vi "calculator.vi"() -> ()   [LabVIEW 2014]
panel:
  in  "stop":bool
  out "String":string
  in  "Cluster":T1
  # "physical keyborad位置設計的有些複雜\n\nF1對應數字鍵1\nF2對應數字鍵2\nF3對應數字鍵3\nF4對應數字鍵4\nF5對應數字鍵5\nF6對應數字鍵6\nF7對應數字鍵7\nF8對應數字鍵8\nF9對應數字鍵9\nF10對應數字鍵0\nF11對符號 . \nPGUP對應加號\nPGON對應減號\nHOME對應乘號\nEND對應除號\nDELETE對應Clear\nENTER對應等號\n\n備註:我使用MSI筆電，按加減乘除時，需搭配shift並按設定鍵兩下才有效果"
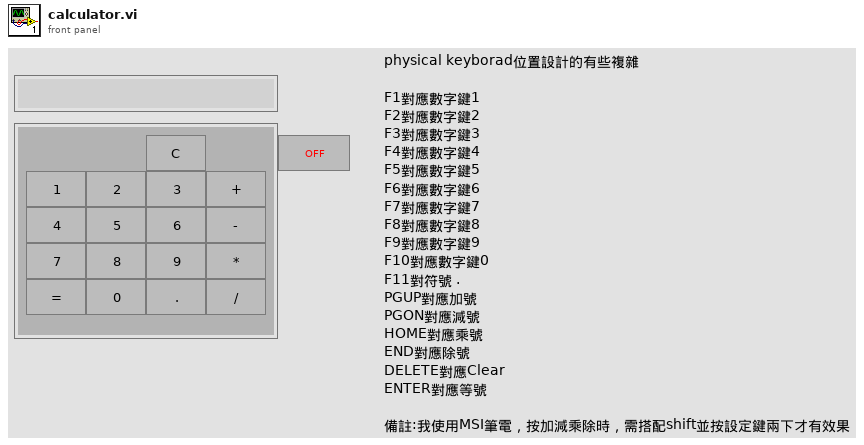
[diagram p1: front panel]
types:
  T1 = cluster{"1":bool, "2":bool, "3":bool, "4":bool, "5":bool, "6":bool, "7":bool, "8":bool, "9":bool, "0":bool, ".":bool, "add":bool, "sub":bool, "mul":bool, "div":bool, "equal":bool, "C":bool}
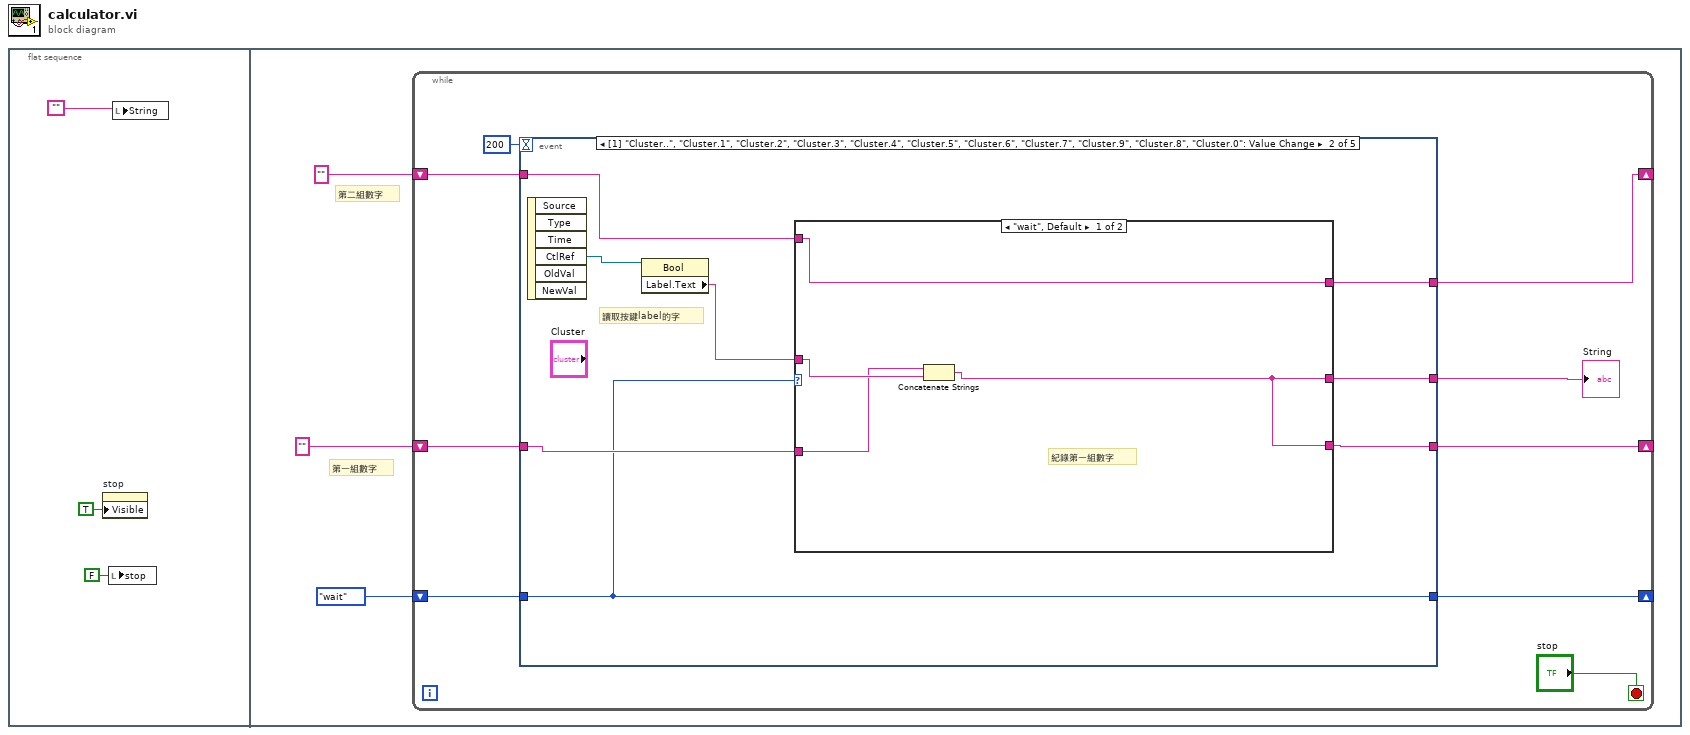
[diagram p0: block diagram]
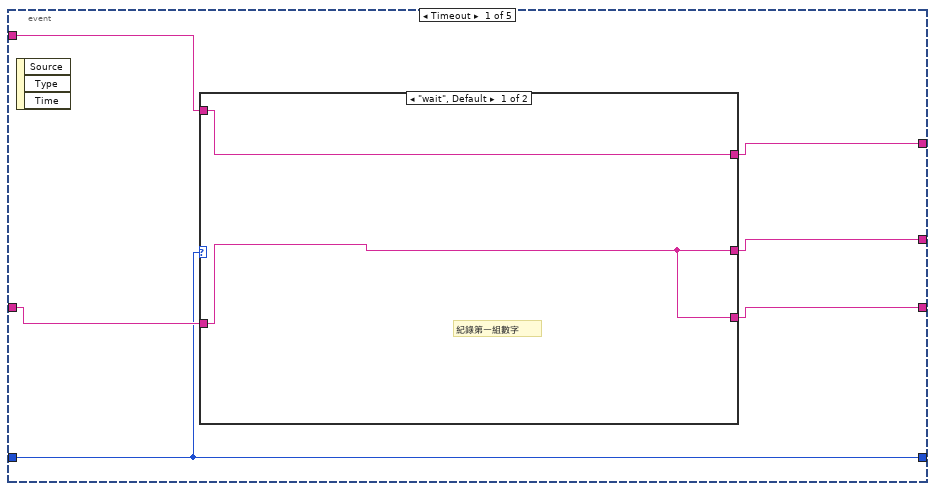
[diagram p2: hidden frame]
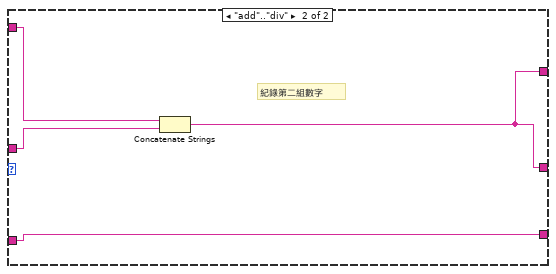
[diagram p4: hidden frame]
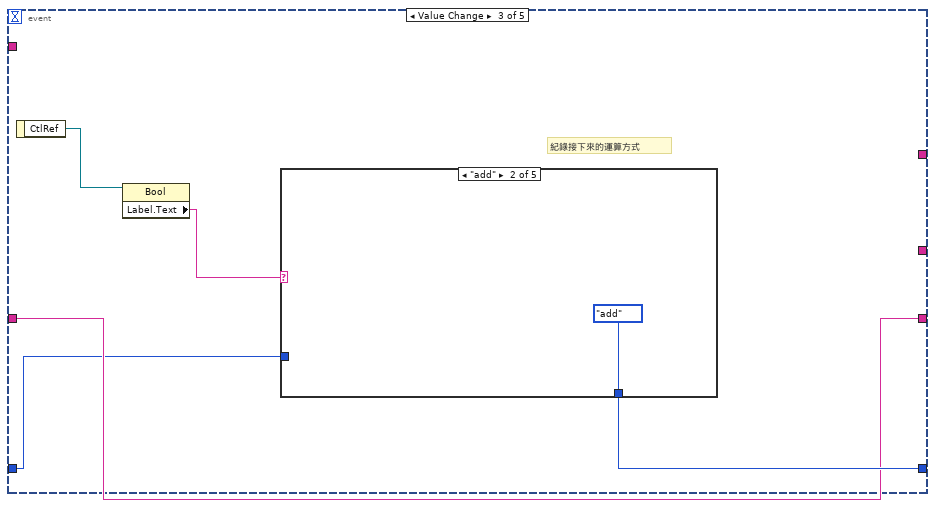
[diagram p5: hidden frame]
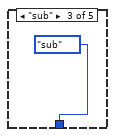
[diagram p7: hidden frame]
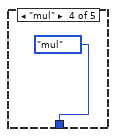
[diagram p8: hidden frame]
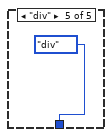
[diagram p9: hidden frame]
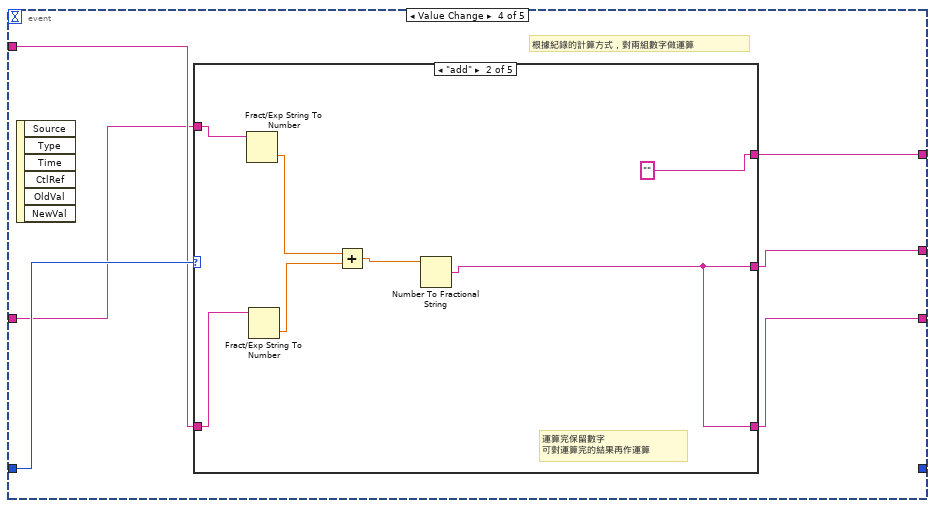
[diagram p10: hidden frame]
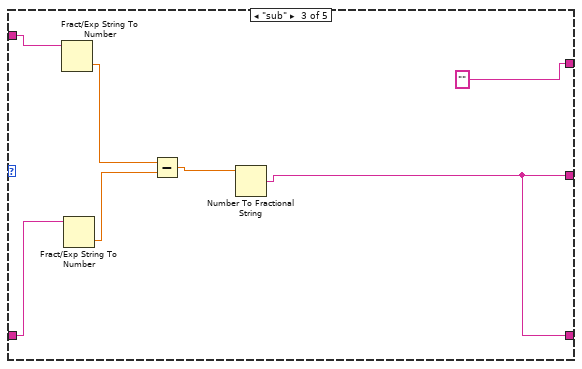
[diagram p12: hidden frame]
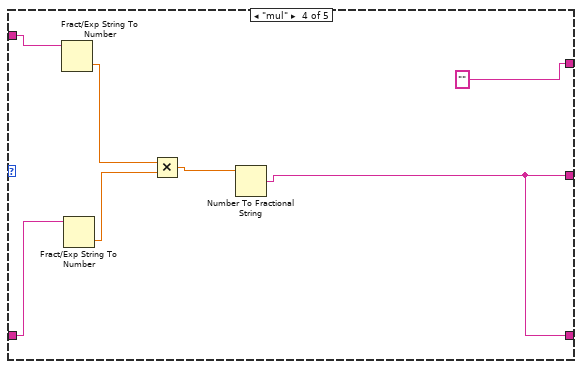
[diagram p13: hidden frame]
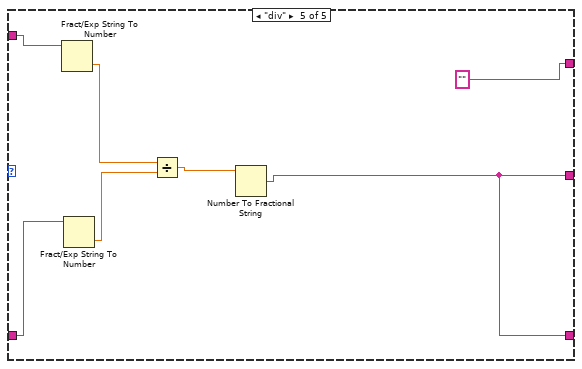
[diagram p14: hidden frame]
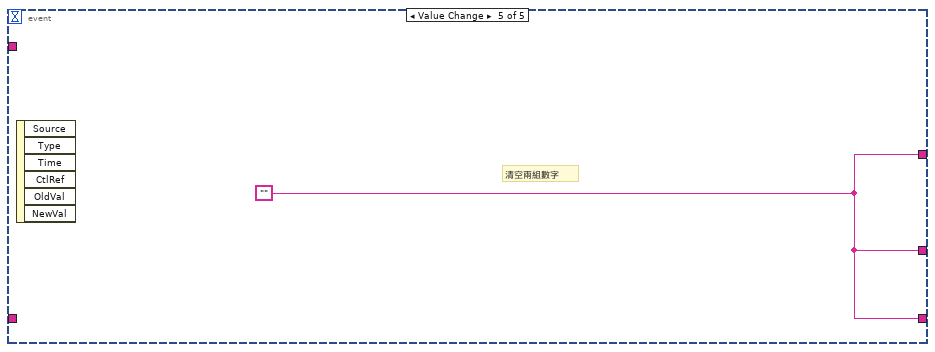
[diagram p15: hidden frame]
diagram:
  n1 = flat-sequence {
    frame #0 {
      n2 = property on="stop" class="Bool (strict)"("Visible"=TRUE) -> ()  [unwired: 2 in, 2 out]
      n3 = local write "stop"(FALSE ("stop")) -> ()
      n4 = local write "String"("") -> ()
    }
    frame #1 {
      # "第二組數字"
      # "第一組數字"
      n5 = while {
        shift-right: [w11] -> _
        shift-left: "" -> [w15]
        shift-right: [w8] -> _
        shift-left: "" -> [w14]
        shift-right: [w12] -> _
        shift-left: enum16{"wait", "add", "sub", "mul", "div"}."wait" -> [w13]
        stop <- "stop" stop-if-true
        n6 = event shown="[1] \"Cluster..\", \"Cluster.1\", \"Cluster.2\", \"Cluster.3\", \"Cluster.4\", \"Cluster.5\", \"Cluster.6\", \"Cluster.7\", \"Cluster.9\", \"Cluster.8\", \"Cluster.0\": Value Change" {
          selector: _ -> [_ _ _ _ _]
          dyn-events: _ -> [_ _ _ _ _]
          timeout: 200 -> [_ _ _ _ _]
          tunnel: w15 -> [w17 w33 _ w53 _]
          tunnel: w14 -> [w21 w32 w43 w52 _]
          tunnel: w13 -> [w16 w30 w42 w57 _]
          tunnel: [w16 w30 w44 _ _] -> w12
          tunnel: [w18 w29 _ w56 w88] -> w11
          tunnel: [w20 w28 _ w54 w88] -> w9
          tunnel: [w19 w27 w43 w55 w88] -> w8
          event Timeout {
            n7 = event-data() -> ()  [unwired: 1 in, 3 out]
            n8 = case shown="\"wait\", Default" w16 {
              tunnel: w17 -> [w23 w24]
              tunnel: w21 -> [w22 w25]
              tunnel: [w23 w24] -> w18
              tunnel: [w22 w24] -> w20
              tunnel: [w22 w25] -> w19
              frame "wait", Default {
                # "紀錄第一組數字"
              }
              frame "add".."div" {
                # "紀錄第二組數字"
              }
            }
          }
          event "Cluster..", "Cluster.1", "Cluster.2", "Cluster.3", "Cluster.4", "Cluster.5", "Cluster.6", "Cluster.7", "Cluster.9", "Cluster.8", "Cluster.0": Value Change {
            # "讀取按鍵label的字"
            n9 = event-data() -> ("CtlRef"=w31:refnum<vi>)  [unwired: 1 in, 5 out]
            n10 = property class="Bool"(reference=w31) -> ("Label.Text"=w26:string)  [unwired: 1 in, 2 out]
            n11 = case shown="\"wait\", Default" w30 {
              tunnel: w33 -> [w34 w40]
              tunnel: w32 -> [w36 w41]
              tunnel: [w34 w38] -> w29
              tunnel: [w35 w38] -> w28
              tunnel: [w35 w41] -> w27
              tunnel: w26 -> [w37 w39]
              frame "wait", Default {
                # "紀錄第一組數字"
                n12 = Concatenate Strings(w36, w37) -> (w35:string)
              }
              frame "add".."div" {
                # "紀錄第二組數字"
                n13 = Concatenate Strings(w40, w39) -> (w38:string)
              }
            }
          }
          event "Cluster.add", "Cluster.sub", "Cluster.mul", "Cluster.div": Value Change {
            # "紀錄接下來的運算方式"
            n14 = event-data() -> ("CtlRef"=w46:refnum<vi>)  [unwired: 1 in]
            n15 = property class="Bool"(reference=w46) -> ("Label.Text"=w45:string)  [unwired: 1 in, 2 out]
            n16 = case shown="\"add\"" w45 {
              tunnel: [w47 enum16{"wait", "add", "sub", "mul", "div"}."add" enum16{"wait", "add", "sub", "mul", "div"}."sub" enum16{"wait", "add", "sub", "mul", "div"}."mul" enum16{"wait", "add", "sub", "mul", "div"}."div"] -> w44
              tunnel: w42 -> [w47 _ _ _ _]
              frame Default {
              }
              frame "add" {
              }
              frame "sub" {
              }
              frame "mul" {
              }
              frame "div" {
              }
            }
          }
          event "Cluster.equal": Value Change {
            # "根據紀錄的計算方式，對兩組數字做運算"
            n17 = event-data() -> ()  [unwired: 1 in, 6 out]
            n18 = case shown="\"add\"" w57 {
              tunnel: w52 -> [w58 w66 w73 w80 w87]
              tunnel: [w58 "" "" "" ""] -> w56
              tunnel: [w59 w60 w67 w74 w81] -> w55
              tunnel: w53 -> [w59 w65 w72 w79 w86]
              tunnel: [w58 w60 w67 w74 w81] -> w54
              frame "wait", Default {
              }
              frame "add" {
                # "運算完保留數字\n可對運算完的結果再作運算"
                n19 = Fract/Exp String To Number(string=w66) -> (number=w63:dbl)  [unwired: 3 in, 1 out]
                n20 = Fract/Exp String To Number(string=w65) -> (number=w64:dbl)  [unwired: 3 in, 1 out]
                n21 = Add(x=w63, y=w64) -> (x+y=w62:dbl)
                n22 = Number To Fractional String(number=w62) -> (F-format string=w60:string)  [unwired: 3 in]
              }
              frame "sub" {
                n23 = Fract/Exp String To Number(string=w73) -> (number=w70:dbl)  [unwired: 3 in, 1 out]
                n24 = Fract/Exp String To Number(string=w72) -> (number=w71:dbl)  [unwired: 3 in, 1 out]
                n25 = Subtract(x=w70, y=w71) -> (x-y=w69:dbl)
                n26 = Number To Fractional String(number=w69) -> (F-format string=w67:string)  [unwired: 3 in]
              }
              frame "mul" {
                n27 = Fract/Exp String To Number(string=w80) -> (number=w77:dbl)  [unwired: 3 in, 1 out]
                n28 = Fract/Exp String To Number(string=w79) -> (number=w78:dbl)  [unwired: 3 in, 1 out]
                n29 = Multiply(x=w77, y=w78) -> (x*y=w76:dbl)
                n30 = Number To Fractional String(number=w76) -> (F-format string=w74:string)  [unwired: 3 in]
              }
              frame "div" {
                n31 = Fract/Exp String To Number(string=w87) -> (number=w84:dbl)  [unwired: 3 in, 1 out]
                n32 = Fract/Exp String To Number(string=w86) -> (number=w85:dbl)  [unwired: 3 in, 1 out]
                n33 = Divide(x=w84, y=w85) -> (x/y=w83:dbl)
                n34 = Number To Fractional String(number=w83) -> (F-format string=w81:string)  [unwired: 3 in]
              }
            }
          }
          event "Cluster.C": Value Change {
            w88 = ""
            # "清空兩組數字"
            n35 = event-data() -> ()  [unwired: 1 in, 6 out]
          }
        }
        "String" <- w9
      }
    }
  }
